vi "KeyControl.vi"() -> ()   [LabVIEW 2010]
uses:
  <vilib>/userDefined/High Color/IMAQdx.ctl
  BotCommands.ctl
  <vilib>/Platform/TimedLoop/XDataNode/XDataNode.xnode
  <vilib>/Platform/TimedLoop/XDataNode/timing_clust.ctl
  <vilib>/Platform/TimedLoop/XDataNode/nitl_modes.ctl
  <vilib>/Platform/TimedLoop/XDataNode/wakeup.ctl
  <vilib>/Utility/inputDevices.llb/closeJoystick.vi
  <vilib>/Utility/inputDevices.llb/joystickAcquire.vi
  <vilib>/Platform/TimedLoop/XDataNode/XDNodeRunTimeDep.lvlib
  <vilib>/vision/driver/NI_Vision_Acquisition_Software.lvlib
panel:
  in  "Camera Name":T1="cam0"
  out "?":T2(plugin-control)
  in  "Target IP":string="10.25.1.100"
  out "Image Error":errorcluster
  out "Rotation (rad/s)":dbl(knob) scale=1.0..-1.0
  out "Speed (m/s)":dbl(knob) scale=-1.0..1.0
  in  "Turn scale":dbl=0.7
  in  "Speed scale":dbl=0.5
  out "Control Error":errorcluster
  in  "stop":bool
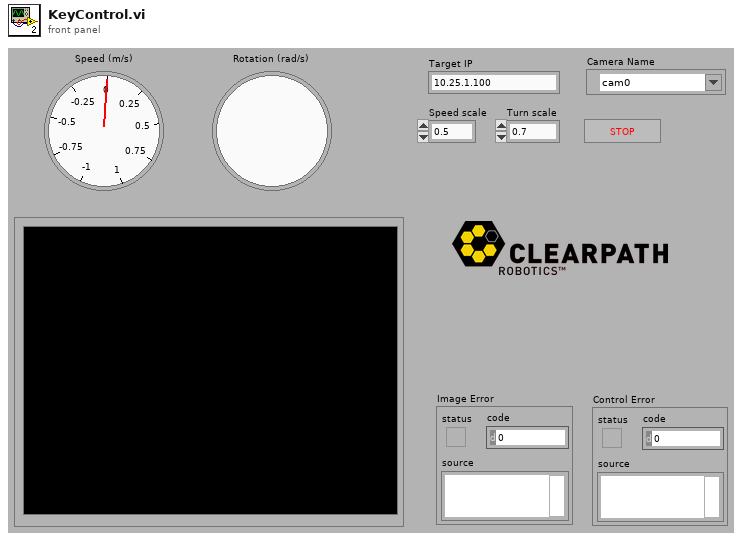
[diagram p1: front panel]
types:
  T1 = typedef "IMAQdx.ctl" = refnum<k21>
  T2 = typedef "IMAQ Image.ctl" = refnum<image>
  T3 = typedef "BotCommands.ctl" = cluster{"Translational":dbl, "Rotational":dbl}
  T4 = typedef "XDNodeRunTimeDep.lvlib/timing_clust.ctl" = cluster{"Expected End [f-1]":u64, "Actual End [f-1]":u64, "Finished Late? [f-1]":bool, "Expected End [i-1]":u64, "Actual End [i-1]":u64, "Finished Late? [i-1]":bool, "Expected Start [i]":u64, "Actual Start [i]":u64, "Expected Start [f]":u64, "Actual Start [f]":u64, "Source Name":string, "Structure Name":string, "Period":i64, "Deadline":i64, "Offset":i64, "Start":i64, "Priority":i32, "Timeout":i32, "Mode":T5, "Wakeup Reason":T6, "Error":errorcluster, "Source Type":string, "Secondary Source Type":string, "Global End Time":u64, "Global Start Time":u64, "Frame Duration":u64, "Iteration Duration":u64, "Assigned CPU":i32, "I/O Scan Engine Mode":u32}
  T5 = typedef "XDNodeRunTimeDep.lvlib/nitl_modes.ctl" = enum32{"No Change", "Process missed periods, maintain original phase", "Discard missed periods, maintain original phase", "Process missed periods, ignore original phase", "Discard missed periods, ignore original phase"}
  T6 = typedef "XDNodeRunTimeDep.lvlib/wakeup.ctl" = enum32{"Normal", "Aborted", "Asynchronous wakeup", "Timing source error", "Timed loop error", "Timeout"}
  T7 = cluster{"X axis":i32, "Y axis":i32, "Z axis":i32, "X axis rotation":i32, "Y axis rotation":i32, "Z axis rotation":i32, "U axis":i32, "V axis":i32}
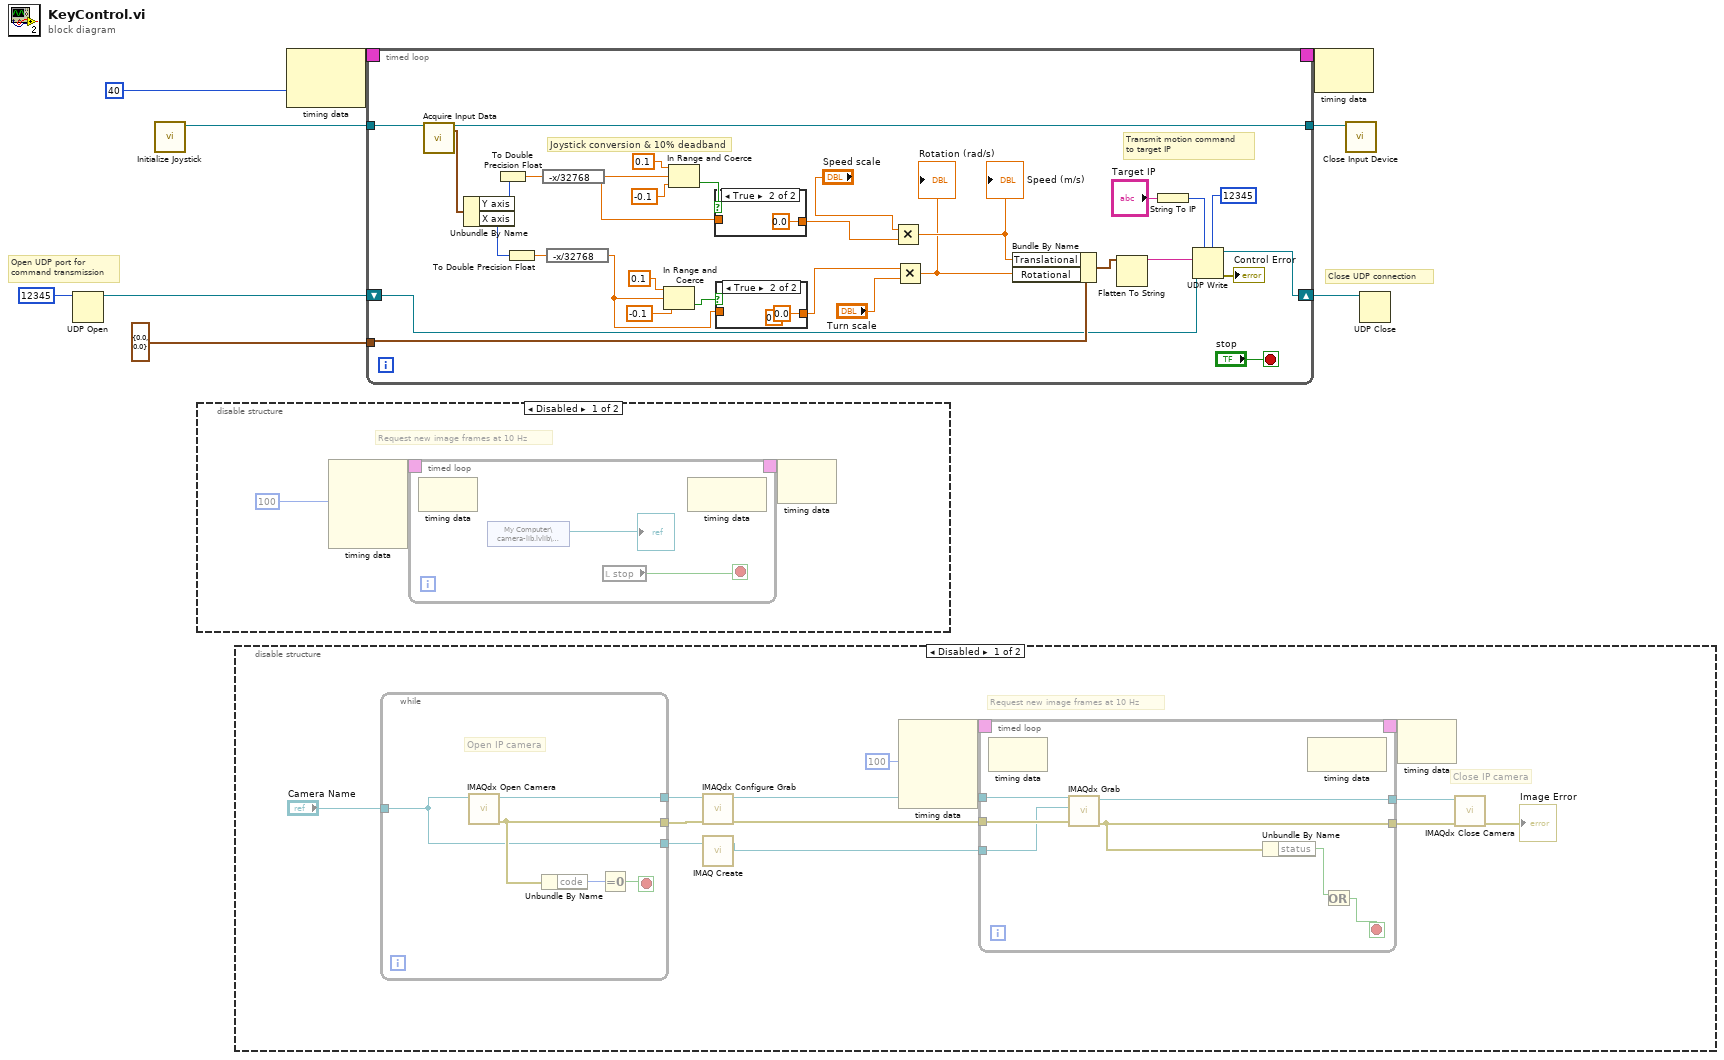
[diagram p0: block diagram]
diagram:
  # "Close UDP connection"
  # "Open UDP port for\ncommand transmission"
  n1 = UDP Open(11:u16 12345 ("remote port")) -> (port=w1:refnum<k16>)  [unwired: 4 in, 2 out]
  n2 = call <vilib>:"Initialize Joystick.vi"() -> ("device ID"=w3:refnum<k1>)  [unwired: 10 in, 1 out]
  n3 = disable-structure shown="Disabled" {
    frame Disabled {
      # "Request new image frames at 10 Hz"
      n4 = node-c288(100) -> (w12:T4)  [unwired: 3 in]
      n5 = timed-loop {
        timing: w12 -> [_]
        timing-out: [_] -> w11
        stop <- w13 stop-if-true
        n6 = node-c288() -> ()  [unwired: 1 in, 1 out]
        n7 = shared-variable "My Computer\\camera-lib.lvlib\\Camera"() -> (→"?":refnum<image>)  [unwired: 1 in, 1 out]
        n8 = local read "stop"() -> (w13:bool)
        n9 = node-c288() -> ()  [unwired: 1 in, 1 out]
      }
      n10 = node-c288(w11) -> ()  [unwired: 1 out]
    }
    frame Enabled {
    }
  }
  n11 = disable-structure shown="Disabled" {
    frame Disabled {
      # "Request new image frames at 10 Hz"
      # "Close IP camera"
      n12 = while {
        tunnel: [w34] -> w25
        tunnel: [w36] -> w27
        tunnel: [w35] -> w26
        tunnel: "Camera Name" -> [w34]
        stop <- w37 stop-if-true
        # "Open IP camera"
        n13 = call <vilib>:"IMAQdx Open Camera.vi"("Session In"=w34) -> ("error out"=w36:errorcluster, "Session Out"=w35:T1)  [unwired: 9 in]
        n14 = Unbundle By Name(w36) -> ("code"=w38:i32)
        n15 = Equal To 0?(x=w38) -> (x = 0?=w37:bool)
      }
      n16 = call <vilib>:"IMAQdx Configure Grab.vi"("error in"=w27, "Session In"=w26) -> ("error out"=w23:errorcluster, "Session Out"=w24:T1)  [unwired: 8 in]
      n17 = call "IMAQ Create"("Image Name"=w25) -> ("New Image"=w22:T2)  [unwired: 4 in, 1 out]
      n18 = node-c288(i64 100 ("Period")) -> (w33:T4)  [unwired: 3 in]
      n19 = timed-loop {
        tunnel: w24 -> [w47]
        tunnel: w23 -> [w46]
        tunnel: w22 -> [w45]
        tunnel: [w41] -> w31
        tunnel: [w44] -> w29
        timing: w33 -> [_]
        timing-out: [_] -> w32
        stop <- w42 stop-if-true
        n20 = node-c288() -> ()  [unwired: 1 in, 1 out]
        n21 = call <vilib>:"IMAQdx Grab.vi"("error in"=w46, "Image In"=w45, "Session In"=w47) -> ("error out"=w41:errorcluster, "Image Out"=w40:T2, "Session Out"=w44:T1)  [unwired: 5 in, 1 out]
        n22 = Unbundle By Name(w41) -> ("status"=w43:bool)
        n23 = node-c288() -> ()  [unwired: 1 in, 1 out]
        n24 = Or(x=w43) -> (y=w39:bool, x .or. y?=w42:bool)
      }
      n25 = node-c288(w32) -> ()  [unwired: 1 out]
      n26 = call <vilib>:"IMAQdx Close Camera.vi"("error in"=w31, "Session In"=w29) -> ("error out"=→"Image Error":errorcluster)  [unwired: 9 in]
    }
    frame Enabled {
    }
  }
  n27 = node-c288(i64 40 ("Period")) -> (w9:T4)  [unwired: 1 in]
  n28 = timed-loop {
    tunnel: w3 -> [w83]
    tunnel: [w82] -> w7
    tunnel: T3 {"Translational"=0.0, "Rotational"=0.0} ("BotCommands") -> [w81]
    shift-right: [w61] -> w5
    shift-left: w1 -> [w64]
    timing: w9 -> [_]
    timing-out: [_] -> w8
    stop <- "stop" stop-if-true
    (unwired) 0.0
    # "Joystick conversion & 10% deadband"
    # "Transmit motion command \nto target IP"
    n29 = call-poly <vilib>:"Acquire Input Data.vi"("device ID"=w83) -> ("device ID"=w82:refnum<k1>, "axis info"=w79:T7)  [unwired: 14 in, 3 out]
    n30 = Unbundle By Name(w79) -> ("Y axis"=w78:i32, "X axis"=w77:i32)
    n31 = To Double Precision Float(number=w78) -> (double precision float=w76:dbl)
    n32 = To Double Precision Float(number=w77) -> (double precision float=w75:dbl)
    n33 = expression code="-x/32768"(w76) -> (w69:dbl)
    n34 = expression code="-x/32768"(w75) -> (w65:dbl)
    n35 = In Range and Coerce(upper limit=0.1, x=w65, lower limit=-0.1 ("upper limit")) -> (In Range?=w66:bool)  [unwired: 1 out]
    n36 = In Range and Coerce(upper limit=0.1, x=w69, lower limit=-0.1 ("upper limit")) -> (In Range?=w72:bool)  [unwired: 1 out]
    n37 = case shown="True" w72 {
      tunnel: [w87 0.0] -> w56
      tunnel: w69 -> [w87 _]
      frame False {
      }
      frame True {
      }
    }
    n38 = case shown="True" w66 {
      tunnel: [w85 0.0] -> w55
      tunnel: w65 -> [w85 _]
      frame False {
      }
      frame True {
      }
    }
    n39 = Multiply(x="Speed scale", y=w56) -> (x*y=w74:dbl)
    "Speed (m/s)" <- w74
    n40 = Multiply(x=w55, y="Turn scale") -> (x*y=w73:dbl)
    "Rotation (rad/s)" <- w73
    n41 = Bundle By Name(cluster=w81, "Translational"=w74, "Rotational"=w73) -> (w80:T3)
    n42 = Flatten To String(anything=w80) -> (data string=w63:string)  [unwired: 2 in, 3 out]
    n43 = String To IP(1:"Target IP") -> (0:w59:u32)
    n44 = UDP Write(address=w59, port or service name=u16 12345, connection ID=w64, data in=w63) -> (error out=→"Control Error":errorcluster, 3:w61:refnum<k16>)  [unwired: 2 in]
  }
  n45 = node-c288(w8) -> ()  [unwired: 1 out]
  n46 = call-poly <vilib>:"Close Input Device.vi"("device ID"=w7) -> ()  [unwired: 9 in, 1 out]
  n47 = UDP Close(connection ID=w5) -> ()  [unwired: 1 in, 2 out]
